vi "AjustesPrevios_2.vi"(8 "error in (no error)":errorcluster) -> (0 "error out":errorcluster, 3 "AjustesPrevios out":refnum<class "AjustesPrevios.lvclass">)   [LabVIEW 2019, in "AjustesPrevios.lvclass"]
uses:
  AjustesPrevios.lvclass
  Prueba04/Control/Slide.ctl
  Prueba04/Prueba04.lvclass
panel:
  in  "Ajuste de amplitud [mV]":T1 scale=0.1..1.5
  out "nivel 2":dbl
  out "voltaje":dbl
  out "nivel":dbl
  in  "seguiente":bool
  # "Verificador"
  # "dB"
  # "V"
  # "Frecuencia"
  # "Hz"
  # "Ajuste Previo 2 : Ajuste Acústico Emisor Multitono"
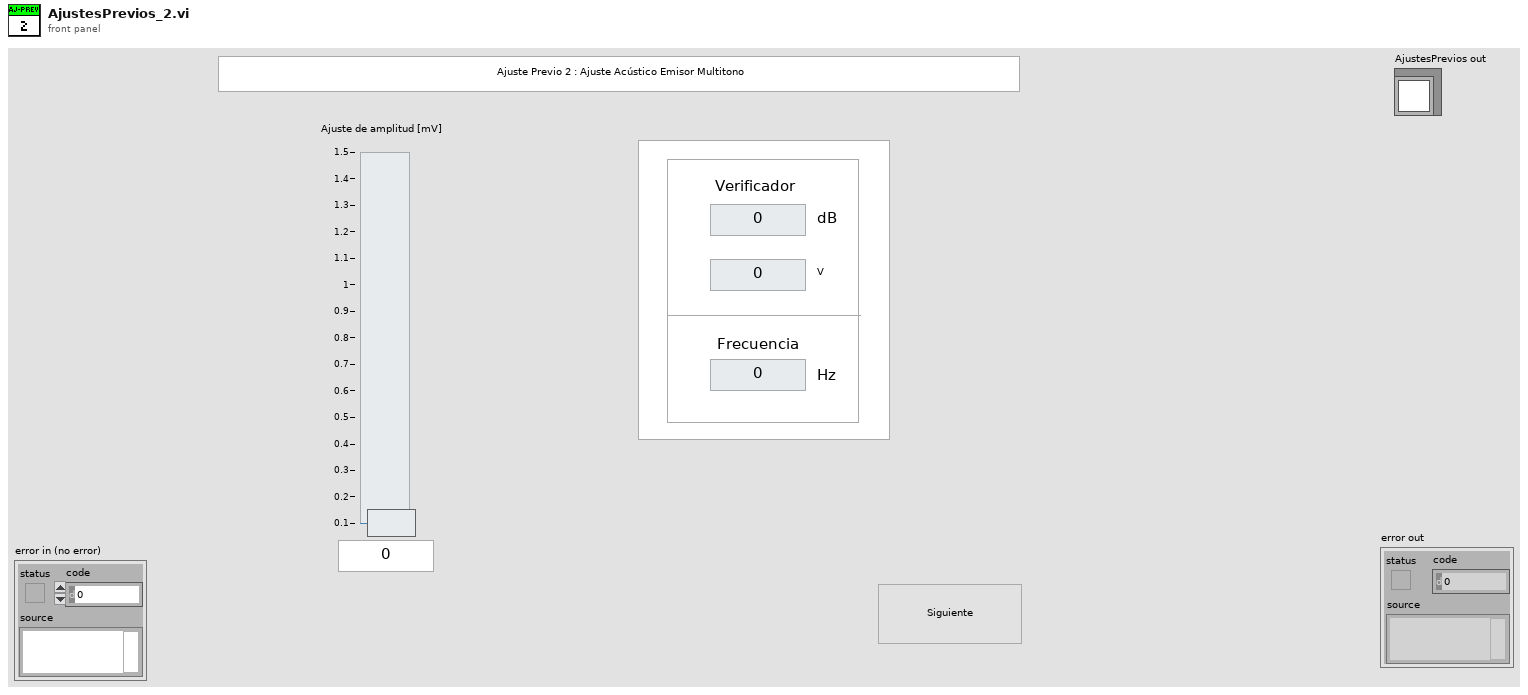
[diagram p1: front panel]
types:
  T1 = typedef "Prueba04.lvclass/Slide.ctl" = dbl
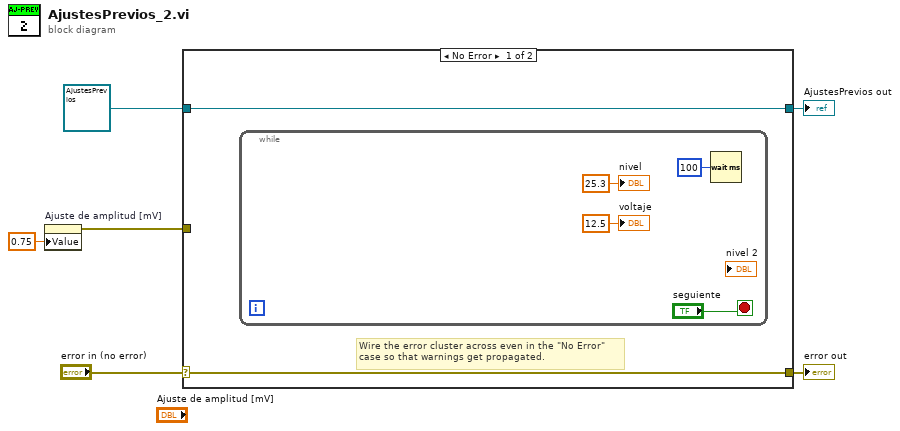
[diagram p0: block diagram]
diagram:
  n1 = property on="Ajuste de amplitud [mV]" class="Slide (strict)"("Value"=T1 0.75 ("Ajuste de amplitud [mV]")) -> (error out=w1:errorcluster)  [unwired: 2 in, 1 out]
  n2 = case shown="No Error" "error in (no error)" {
    selector: "error in (no error)" -> [w7 w14]
    tunnel: [w7 w14] -> w5
    tunnel: [w8 w13] -> w3
    tunnel: refnum<class "AjustesPrevios.lvclass"> refnum ("AjustesPrevios in") -> [w8 w13]
    tunnel: w1 -> [_ _]
    frame No Error {
      # "Wire the error cluster across even in the \"No Error\"\ncase so that warnings get propagated."
      n3 = while {
        stop <- "seguiente" stop-if-true
        n4 = Wait (ms)(milliseconds to wait=u32 100) -> ()  [unwired: 1 out]
        "voltaje" <- 12.5 ("voltaje")
        "nivel" <- 25.3 ("nivel")
      }
    }
    frame Error {
    }
  }
  "error out" <- w5
  "AjustesPrevios out" <- w3
